vi "Lab4_Ex1.vi"() -> ()   [LabVIEW 2019]
uses:
  Ex1_States.ctl
  Ex1_ErrorStatus.ctl
  <vilib>/Utility/file.llb/Write Delimited Spreadsheet (string).vi
panel:
  in  "file path (dialog if empty)":path
  in  "OK Button":bool
  out "ErrorIndicator":string
  in  "Age":u8
  in  "First name":string="Firstname"
  in  "Last name":string="Lastname"
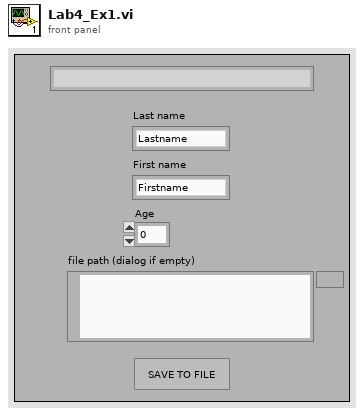
[diagram p1: front panel]
types:
  T1 = typedef "Ex1_ErrorStatus.ctl" = enum16{"NoError", "IllegalAgeError", "EmptyFirstNameError", "EmptyLastNameError", "MultipleErrors"}
  T2 = typedef "Ex1_States.ctl" = enum16{"Start", "CheckErrors", "DisplayErrorMsg", "CkeckButtonPress", "WriteToFile"}
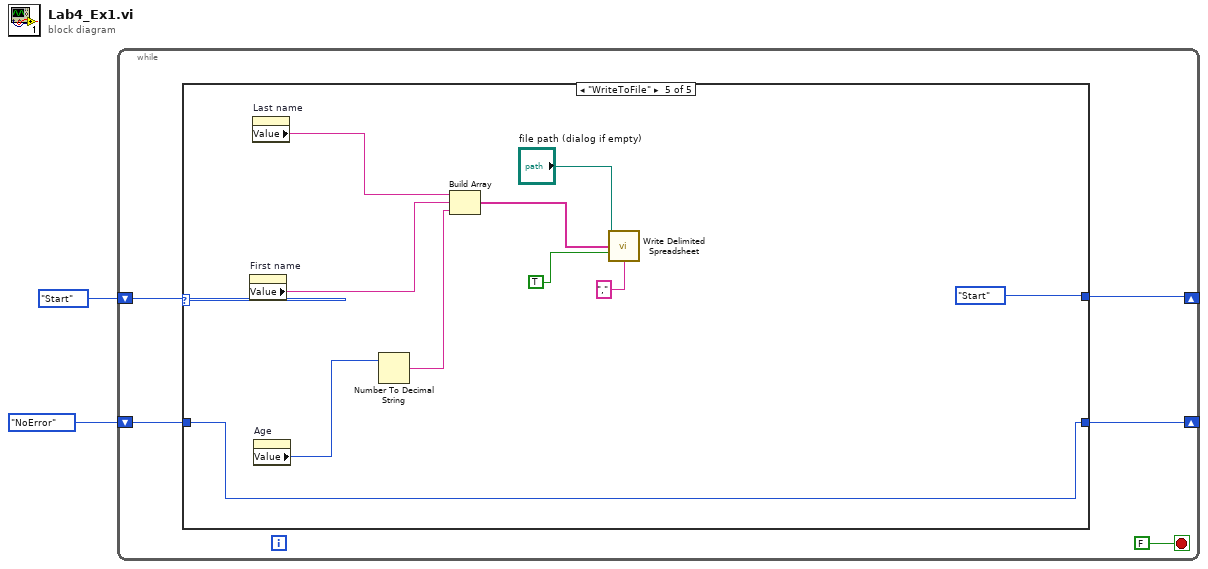
[diagram p0: block diagram]
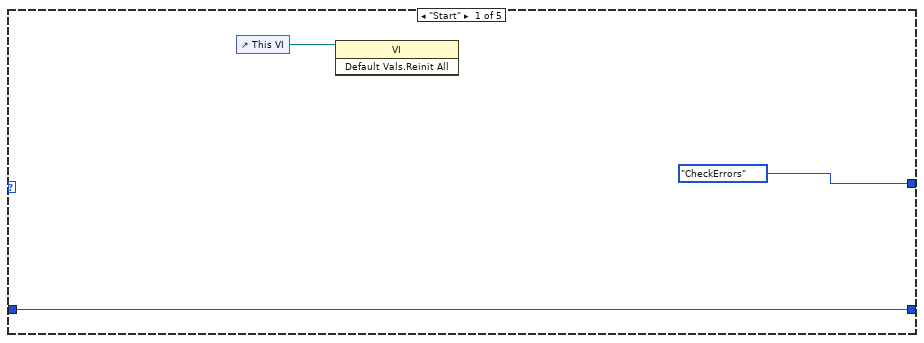
[diagram p2: hidden frame]
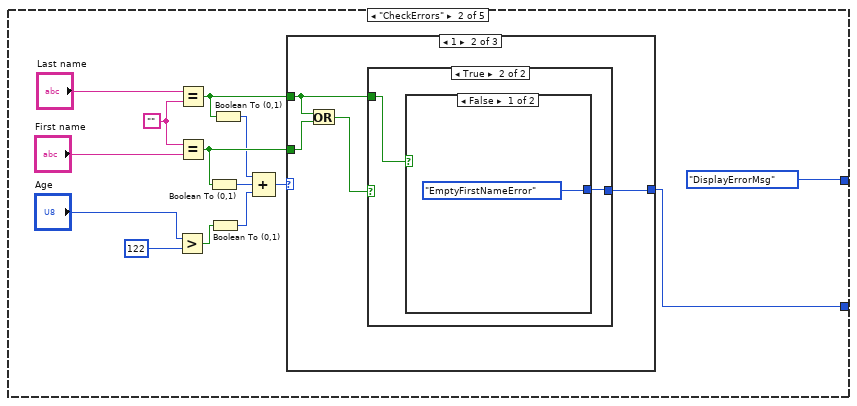
[diagram p3: hidden frame]
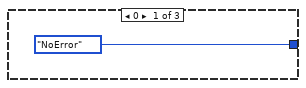
[diagram p4: hidden frame]
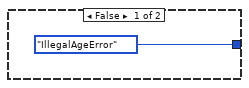
[diagram p5: hidden frame]
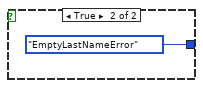
[diagram p6: hidden frame]
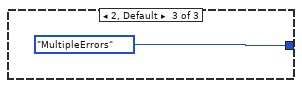
[diagram p7: hidden frame]
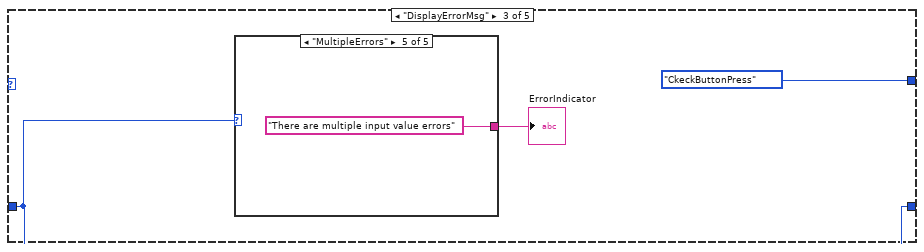
[diagram p8: hidden frame]
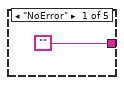
[diagram p9: hidden frame]
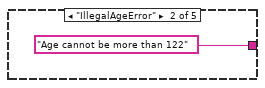
[diagram p10: hidden frame]
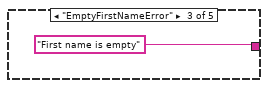
[diagram p11: hidden frame]
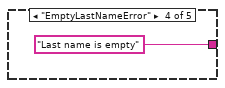
[diagram p12: hidden frame]
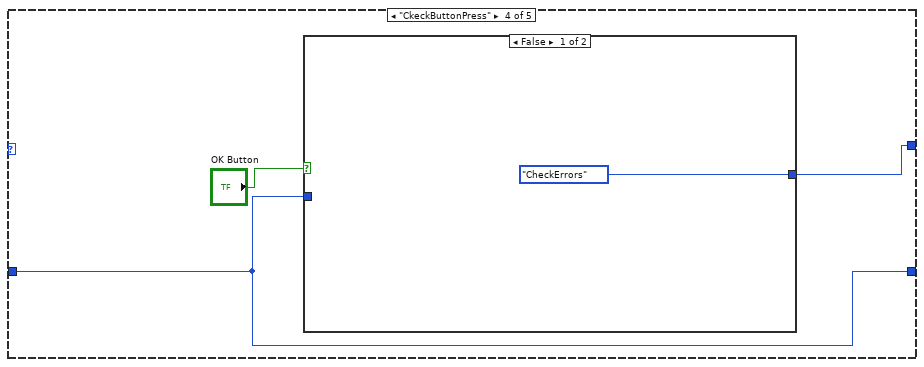
[diagram p13: hidden frame]
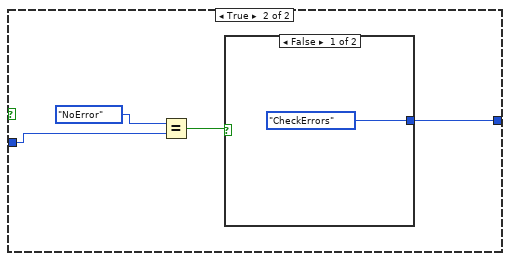
[diagram p14: hidden frame]
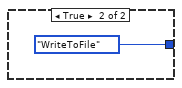
[diagram p15: hidden frame]
diagram:
  n1 = while {
    shift-right: [w6] -> _
    shift-left: Ex1_States."Start" -> [w7]
    shift-right: [w4] -> _
    shift-left: Ex1_ErrorStatus."NoError" -> [w5]
    stop <- FALSE stop-if-true
    n2 = case shown="\"WriteToFile\"" w7 {
      tunnel: [Ex1_States."CheckErrors" Ex1_States."DisplayErrorMsg" Ex1_States."CkeckButtonPress" w45 Ex1_States."Start"] -> w6
      tunnel: w5 -> [w8 _ w36 w44 w56]
      tunnel: [w8 w12 w36 w44 w56] -> w4
      frame "Start" {
        n3 = control-ref of="This VI"() -> (w10:refnum<vi>)
        n4 = invoke class="VI" method="Default Vals.Reinit All"(reference=w10) -> ()  [unwired: 2 in, 3 out]
      }
      frame "CheckErrors" {
        w23 = ""
        n5 = Greater?(x="Age", y=122) -> (0:w17:bool)
        n6 = Equal?(x="Last name", y=w23) -> (x = y?=w19:bool)
        n7 = Equal?(x=w23, y="First name") -> (x = y?=w18:bool)
        n8 = Boolean To (0,1)(Boolean=w18) -> (0, 1=w14:i16)
        n9 = Boolean To (0,1)(Boolean=w17) -> (0, 1=w13:i16)
        n10 = Boolean To (0,1)(Boolean=w19) -> (0, 1=w15:i16)
        n11 = Compound Arithmetic op=ADD(w15, w14, w13) -> (w16:i16)
        n12 = case shown="1" w16 {
          tunnel: [Ex1_ErrorStatus."NoError" w28 Ex1_ErrorStatus."MultipleErrors"] -> w12
          tunnel: w19 -> [_ w27 _]
          tunnel: w18 -> [_ w26 _]
          frame 0 {
          }
          frame 1 {
            n13 = Or(x=w27, y=w26) -> (x .or. y?=w29:bool)
            n14 = case shown="True" w29 {
              tunnel: [Ex1_ErrorStatus."IllegalAgeError" w31] -> w28
              tunnel: w27 -> [_ w32]
              frame False {
              }
              frame True {
                n15 = case shown="False" w32 {
                  tunnel: [Ex1_ErrorStatus."EmptyFirstNameError" Ex1_ErrorStatus."EmptyLastNameError"] -> w31
                  frame False {
                  }
                  frame True {
                  }
                }
              }
            }
          }
          frame 2, Default {
          }
        }
      }
      frame "DisplayErrorMsg" {
        n16 = case shown="\"MultipleErrors\"" w36 {
          tunnel: ["" "Age cannot be more than 122" "First name is empty" "Last name is empty" "There are multiple input value errors"] -> w38
          frame "NoError" {
          }
          frame "IllegalAgeError" {
          }
          frame "EmptyFirstNameError" {
          }
          frame "EmptyLastNameError" {
          }
          frame "MultipleErrors" {
          }
        }
        "ErrorIndicator" <- w38
      }
      frame "CkeckButtonPress" {
        n17 = case shown="False" "OK Button" {
          tunnel: w44 -> [_ w51]
          tunnel: [Ex1_States."CheckErrors" w48] -> w45
          frame False {
          }
          frame True {
            n18 = Equal?(x=Ex1_ErrorStatus."NoError", y=w51) -> (x = y?=w49:bool)
            n19 = case shown="False" w49 {
              tunnel: [Ex1_States."CheckErrors" Ex1_States."WriteToFile"] -> w48
              frame False {
              }
              frame True {
              }
            }
          }
        }
      }
      frame "WriteToFile" {
        n20 = property on="First name" class="Str"() -> ("Value"=w60:string)  [unwired: 2 in, 2 out]
        n21 = property on="Last name" class="Str"() -> ("Value"=w61:string)  [unwired: 2 in, 2 out]
        n22 = property on="Age" class="DigNum (strict)"() -> ("Value"=w63:u8)  [unwired: 2 in, 2 out]
        n23 = Number To Decimal String(number=w63) -> (decimal integer string=w59:string)  [unwired: 1 in]
        n24 = Build Array(w61, w60, w59) -> (w58:string[])
        n25 = call-poly <vilib>:"Write Delimited Spreadsheet.vi"("file path (dialog if empty)"="file path (dialog if empty)", "1D data"=w58, "append to file? (new file:F)"=TRUE, "delimiter (\\t)"=",") -> ()  [unwired: 10 in, 2 out]
      }
    }
  }
